vi "Send.vi"(9 "Nest Alias":string, 10 "Nest Actor":refnum<class "LVCAM.lvclass">) -> (3 "LVCAM Create Nest Msg out":refnum<class "LVCAM Create Nest Msg.lvclass">)   [LabVIEW 2021, in "LVCAM Create Nest.lvlib" / "LVCAM Create Nest Msg.lvclass"]
uses:
  LVCAM Create Nest Msg.lvclass
  LVCAM/LVCAM/LVCAM.lvclass
  LVCAM Create Nest Msg.lvclass/LVCAM Create Nest Msg.ctl
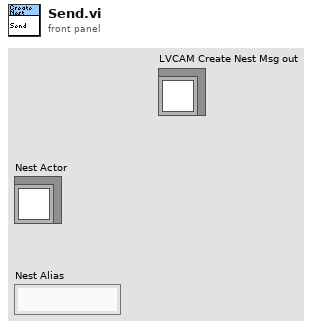
[diagram p1: front panel]
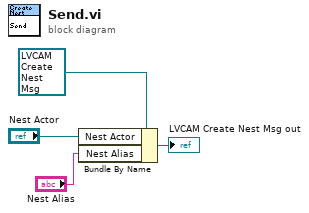
[diagram p0: block diagram]
diagram:
  n1 = Bundle By Name(cluster=refnum<class "LVCAM Create Nest Msg.lvclass"> refnum ("Create Msg in"), "Nest Actor"="Nest Actor", "Nest Alias"="Nest Alias") -> (→"LVCAM Create Nest Msg out":refnum<class "LVCAM Create Nest Msg.lvclass">)
